vi "Lab3_MotorPID_Tutorial.vi"() -> ()   [LabVIEW 2017]
uses:
  <vilib>/myRIO/Common/Instrument Driver Framework/myRIO v1.0/UART/vis/myRIO v1.0 Close UART.vi
  <vilib>/addons/control/pid/pid.llb/PID (DBL).vi
  <vilib>/myRIO/Common/Instrument Driver Framework/Utilities/vis/FPGA Ref Manager.vi
  <vilib>/myRIO/Common/Instrument Driver Framework/myRIO v1.0/myRIO v1.0 Reset FPGA.vi
  <vilib>/myRIO/Common/Instrument Driver Framework/myRIO v1.0/IRQ/vis/myRIO v1.0 IRQ Info FGV.vi
  <vilib>/myRIO/Common/Instrument Driver Framework/myRIO v1.0/IRQ/vis/myRIO v1.0 Timer IRQ Info FGV.vi
  <vilib>/myRIO/Common/Instrument Driver Framework/myRIO v1.0/IRQ/vis/myRIO v1.0 ISR Agent.vi
  <vilib>/addons/control/pid/NI_PID_pid.lvlib
  <vilib>/myRIO/Instrument Drivers/Utilities/Utilities.lvlib
panel:
  in  "output range":cluster{"output high":dbl, "output low":dbl}={"output high"=100.0, "output low"=-100.0} {"output low" format="%.2f"; "output high" format="%.2f"}
  out "output":dbl format="%.2f"
  out "Waveform Chart":dynamicdata(graph)
  in  "setpoint":dbl(slide) scale=-360.0..360.0
  in  "PID gains":T1={"proportional gain (Kc)"=1.0, "integral time (Ti, min)"=0.01, "derivative time (Td, min)"=0.0} {"derivative time (Td, min)" format="%.3f"; "integral time (Ti, min)" format="%.3f"; "proportional gain (Kc)" format="%.3f"}
  in  "stop":bool
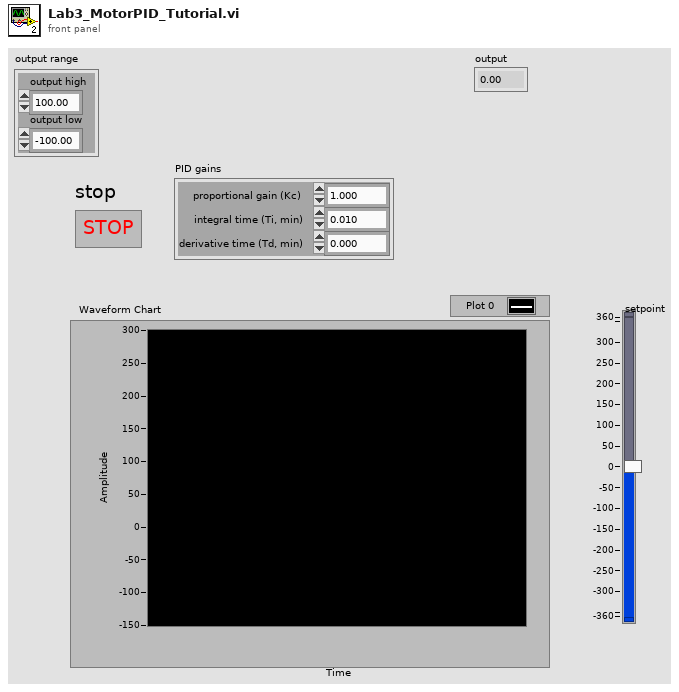
[diagram p1: front panel]
types:
  T1 = cluster{"proportional gain (Kc)":dbl, "integral time (Ti, min)":dbl, "derivative time (Td, min)":dbl}
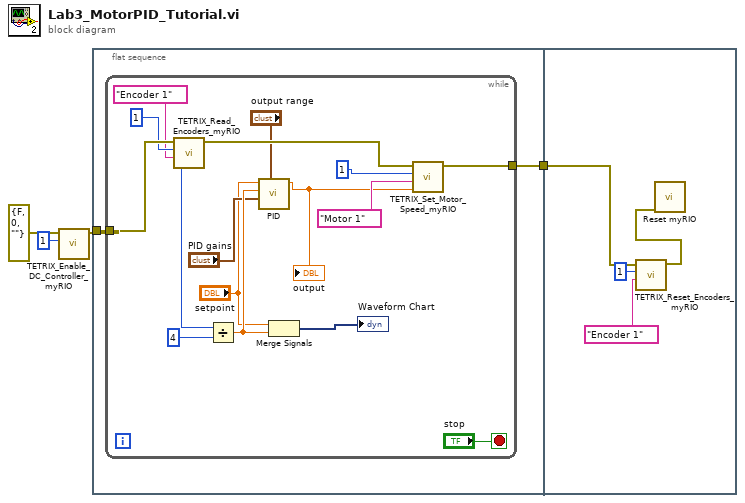
[diagram p0: block diagram]
diagram:
  n1 = call <vilib>:"TETRIX_Enable_DC_Controller_myRIO.vi"("Controller ID#  (I2C Address)"=u8 1, "Error/Flow In"=errorcluster {"status"=FALSE, "code"=0, "source"=""} ("error constant")) -> ("Error/Flow Out"=w3:errorcluster)  [unwired: 5 in]
  n2 = flat-sequence {
    tunnel: w3 -> [w6]
    tunnel: [w5] -> w4
    tunnel: w4 -> [w26]
    frame #0 {
      n3 = while {
        tunnel: w6 -> [w21]
        tunnel: [w12] -> w5
        stop <- "stop" stop-if-true
        n4 = call <vilib>:"TETRIX_Read_Encoders_myRIO.vi"("Select Encoder"="Encoder 1", "Controller ID#  (I2C Address)"=u8 1, "Error/Flow In"=w21) -> ("Error/Flow Out"=w11:errorcluster, "Encoder Output"=w18:i32)  [unwired: 3 in]
        n5 = Divide(x=w18, y=4) -> (x/y=w16:dbl)
        n6 = call-poly <vilib>:"PID.vi"("output range"="output range", "PID gains"="PID gains", "process variable"=w16, "setpoint"="setpoint") -> ("output"=w9:dbl)  [unwired: 6 in, 1 out]
        "output" <- w9
        n7 = Merge Signals("setpoint", w16) -> (→"Waveform Chart":dynamicdata)
        n8 = call <vilib>:"TETRIX_Set_Motor_Speed_myRIO.vi"("Constant Speed (Degrees per second). Sign (+/-)  sets direction."=w9, "Select Channel"="Motor 1", "Controller ID#  (I2C Address)"=u8 1, "Error/Flow In"=w11) -> ("Error/Flow Out"=w12:errorcluster)  [unwired: 3 in]
      }
    }
    frame #1 {
      n9 = call <vilib>:"TETRIX_Reset_Encoders_myRIO.vi"("Select Encoder"="Encoder 1", "Controller ID#  (I2C Address)"=u8 1, "Error/Flow In"=w26) -> ("Error/Flow Out"=w25:errorcluster)  [unwired: 4 in]
      n10 = call <vilib>:"Reset myRIO.vi"("error in (no error)"=w25) -> ()  [unwired: 10 in, 1 out]
    }
  }
